vi "OpenXL_WorkSheet.vi"(6 "Sheet":variant, 8 "error in (no error)":errorcluster, 11 "Refnum Cluster In":T1) -> (0 "error out":errorcluster, 3 "Refnum Cluster Out":T2)   [LabVIEW 2017, in "excel_configuration.lvlib"]
doc: "Opens a worksheet of the current workbook. Sheet accepts either the worksheet index or its name."
uses:
  excel_configuration.lvlib
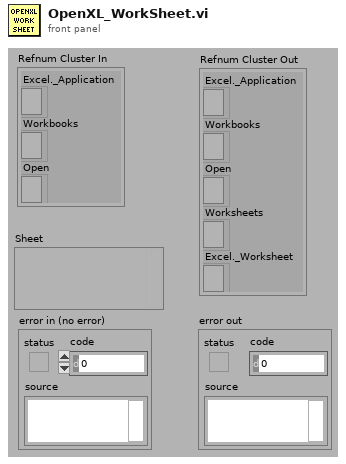
[diagram p1: front panel]
types:
  T1 = cluster{"Excel._Application":refnum<k7>, "Workbooks":refnum<k7>, "Open":refnum<k7>}
  T2 = cluster{"Excel._Application":refnum<k7>, "Workbooks":refnum<k7>, "Open":refnum<k7>, "Worksheets":refnum<k7>, "Excel._Worksheet":refnum<k7>}
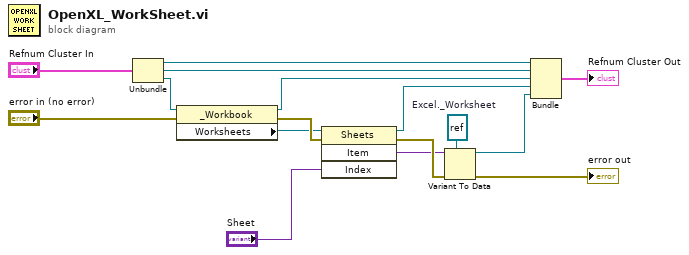
[diagram p0: block diagram]
diagram:
  w10 = refnum<k7> refnum  # Excel._Worksheet
  n1 = Unbundle("Refnum Cluster In") -> ("Excel._Application"=w5:refnum<k7>, "Workbooks"=w6:refnum<k7>, "Open"=w4:refnum<k7>)
  n2 = property class="_Workbook"(reference=w4, error in="error in (no error)") -> (reference out=w14:refnum<k7>, error out=w11:errorcluster, "Worksheets"=w8:refnum<k7>)
  n3 = invoke class="Sheets" method="Item"(reference=w8, error in=w11, "Index"="Sheet") -> (reference out=w15:refnum<k7>, error out=w12:errorcluster, "Item"=w9:variant)  [unwired: 1 in, 1 out]
  n4 = Variant To Data(error in=w12, type=w10, Variant=w9) -> (data=w16:refnum<k7>, error out=→"error out":errorcluster)
  n5 = Bundle("Excel._Application"=w5, "Workbooks"=w6, "Open"=w14, "Worksheets"=w15, "Excel._Worksheet"=w16) -> (→"Refnum Cluster Out":T2)  [unwired: 1 in]
